vi "Actor Core.vi"(8 "error in":errorcluster, 11 "Import Export in":refnum<class "Import Export SQL.lvclass">) -> (0 "error out":errorcluster, 3 "Actor out":refnum<class "Actor.lvclass">)   [LabVIEW 2023, in "Data Analysis.lvlib" / "Import Export SQL.lvlib" / "Import Export SQL.lvclass"]
doc: "(<B>Filename</B>: Actor Framework.lvlib:Actor.lvclass:Actor Core.vi)\n\nReceives messages to the actor, reacts to them, and initiates any error handling that may shut the actor down.\n\nDescendant classes may override this VI to append parallel tasks for the actor to complete while it handles messages. Overrides use the Call Parent Class Method node."
uses:
  Import Export SQL.lvclass
  C:/Program Files/National Instruments/LabVIEW 2023/vi.lib/ActorFramework/Actor/Actor.lvclass
  <vilib>/ActorFramework/Actor/Actor.lvclass
  Import Export SQL.lvclass/Import Export SQL.ctl
  <vilib>/ActorFramework/Actor/Actor.lvclass/Actor.ctl
  <vilib>/ActorFramework/Message Enqueuer/Message Enqueuer.lvclass/Message Enqueuer.ctl
  Subpanel-Abstract Messages/Insert SP Msg/Insert SP Msg.lvclass/Insert SP Msg.ctl
  Import Export SQL Messages/Write Schema Name Msg/Write Schema Name Msg.lvclass/Write Schema Name Msg.ctl
  Import Export SQL Messages/Export SQL Msg/Export SQL Msg.lvclass/Export SQL Msg.ctl
  Import Export SQL Messages/Import SQL Msg/Import SQL Msg.lvclass/Import SQL Msg.ctl
  <vilib>/ActorFramework/Message Enqueuer/Init from Existing Queue.vi
  <vilib>/ActorFramework/Message Enqueuer/Enqueue.vi
  Subpanel-Abstract Messages/Insert SP Msg/Insert SP Msg.lvclass
  C:/Program Files/National Instruments/LabVIEW 2023/vi.lib/ActorFramework/Message/Message.lvclass
  Import Export SQL Messages/Show the Schemas Msg/Show the Schemas Msg.lvclass
  Import Export SQL Messages/Write Schema Name Msg/Write Schema Name Msg.lvclass
  Import Export SQL Messages/Export SQL Msg/Export SQL Msg.lvclass
  Import Export SQL Messages/Import SQL Msg/Import SQL Msg.lvclass
  <vilib>/ActorFramework/Message Priority Queue/Priority Enqueue.vi
  <vilib>/ActorFramework/Message Enqueuer/Message Enqueuer.lvclass
  Subpanel-Abstract/Subpanel-Abstract.lvclass
  D:/eDCU LTT/VT LTT Project/Source Code/Data Analysis/Subpanel-Abstract/Subpanel-Abstract.lvclass
  D:/eDCU LTT/VT LTT Project/Source Code/Data Analysis/Import Export SQL/Import Export/Import Export SQL.lvclass
panel:
  out "Status":string
  in  "Tab Control":enum32{"Import", "Export"}(tab)
  in  "Select the test log file to be imported(.sql)":path
  in  "Import Schema Name":string(combo) caption="Schema Name"
  in  "Import SQL":bool
  in  "Select the Folder":path
  in  "Export Schema Name":string(combo) caption="Test Log Name"
  in  "Export SQL":bool
  in  "Schema Names":string(combo)
  in  "Stop":bool
  # "One Combo Box- Show all the Tables for Selected Schema.\n2. Export Option Enable FE, FF Actor to"
  # "Export Data"
  # "*All filters are applicable here"
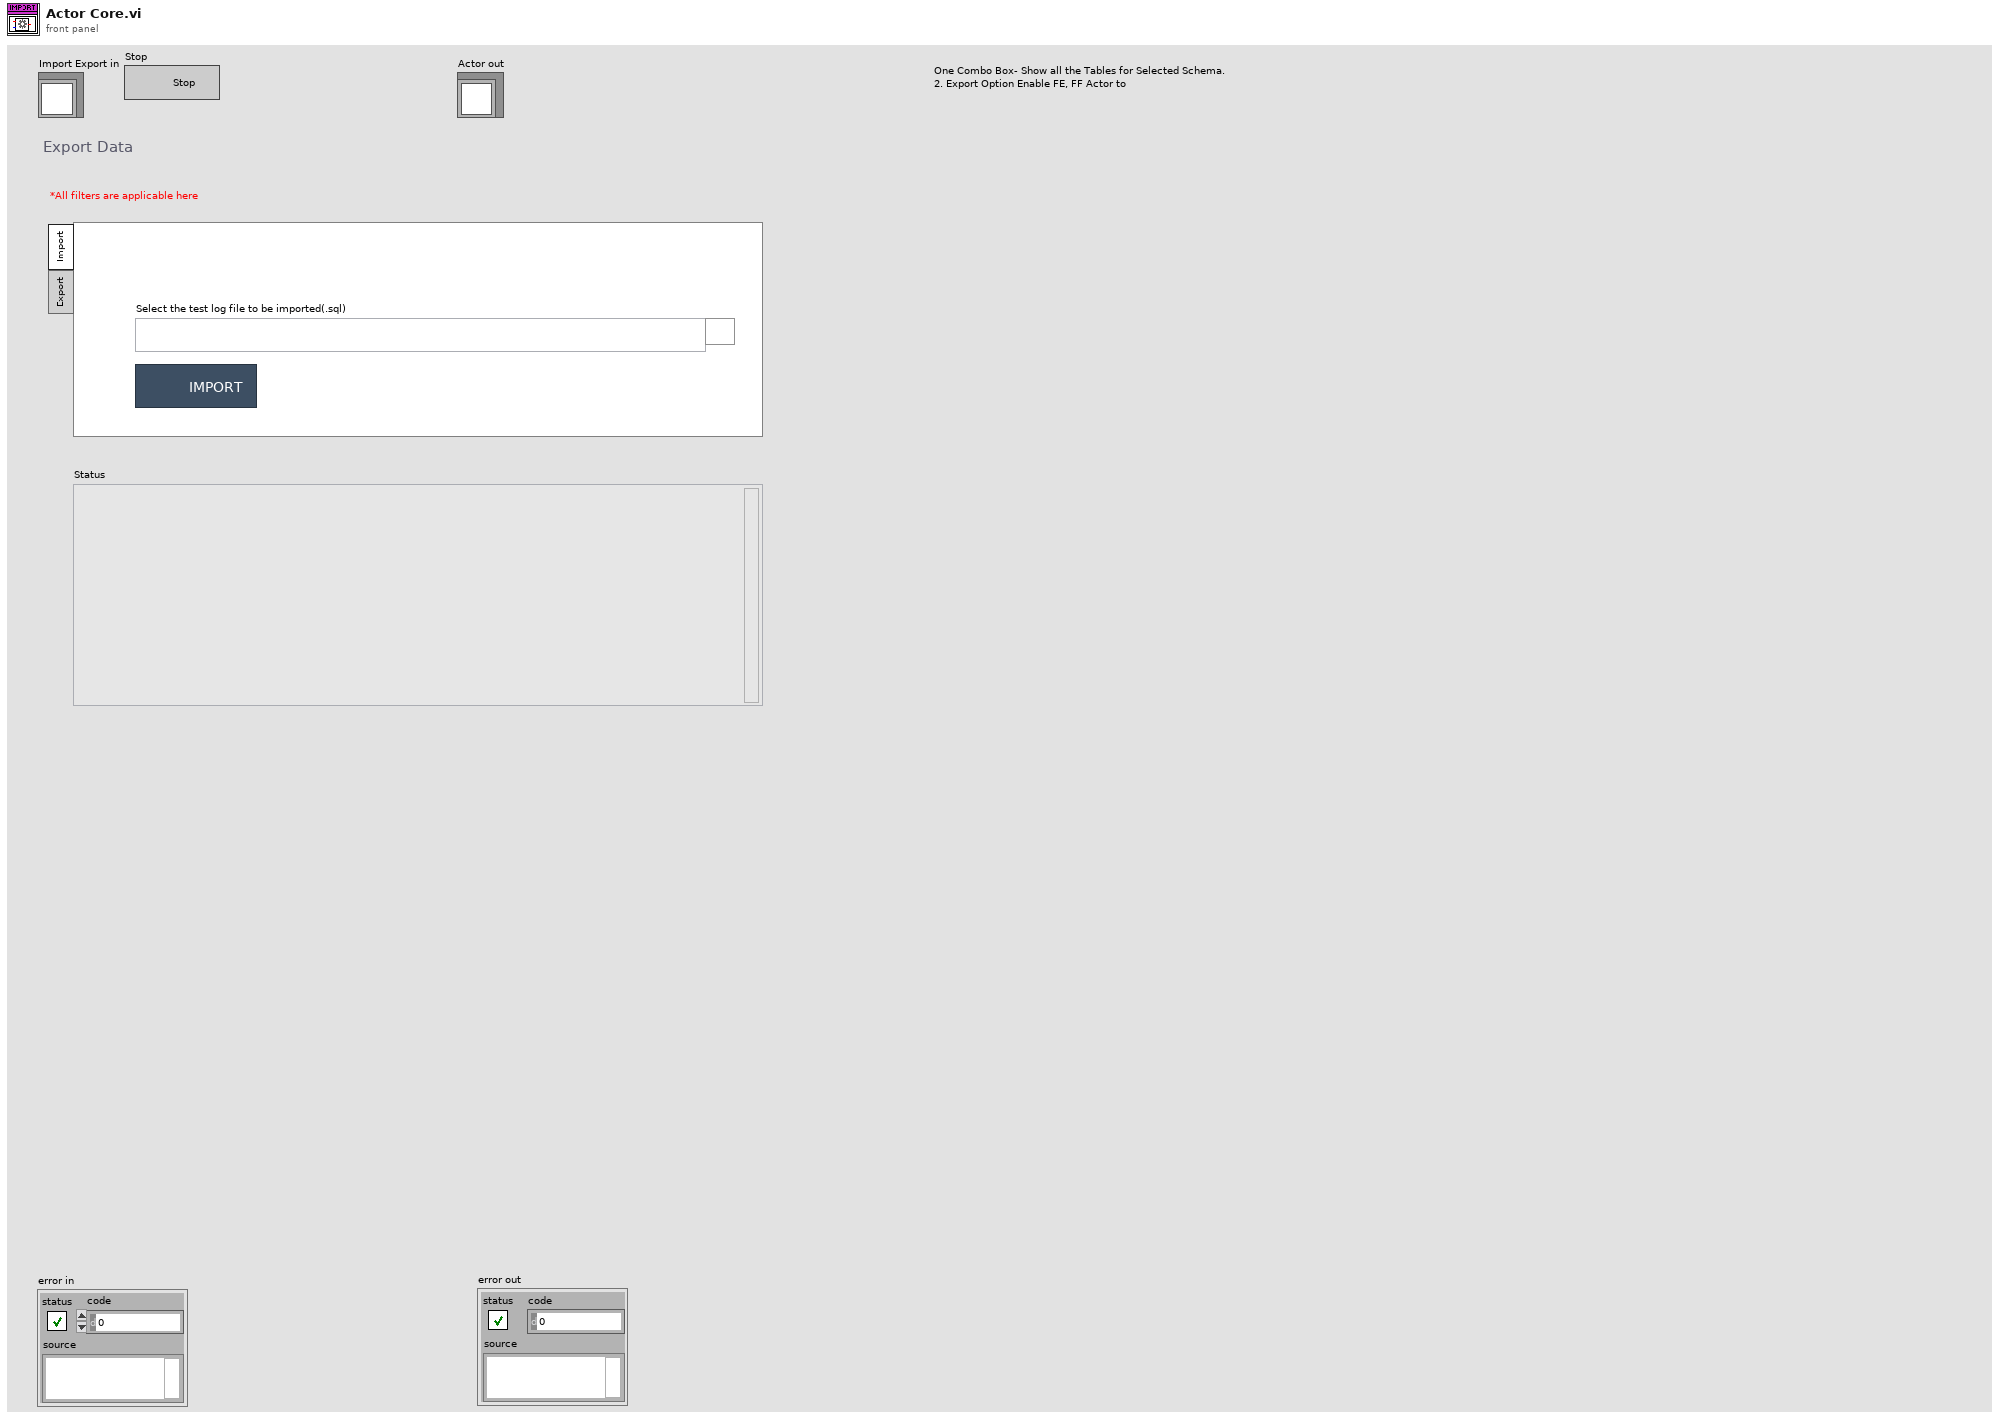
[diagram p1: front panel]
types:
  T1 = cluster{"Schema":string, "Save File Path":path, "Script File Path":path}
  T2 = cluster{"Schema Name":string, "Dump File Path":path, "Script Path":path}
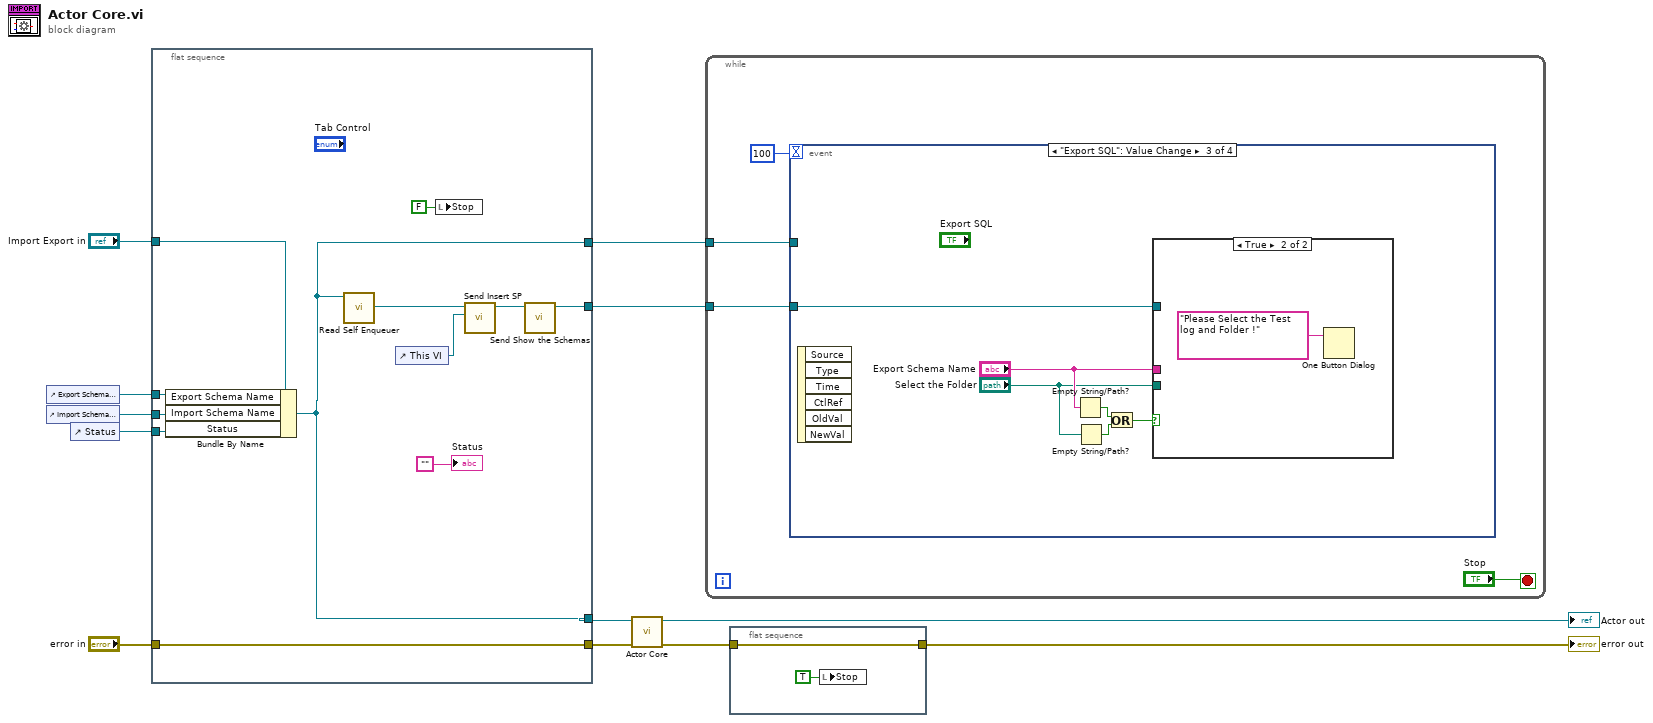
[diagram p0: block diagram]
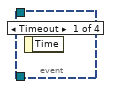
[diagram p2: hidden frame]
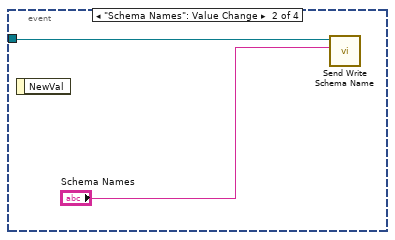
[diagram p3: hidden frame]
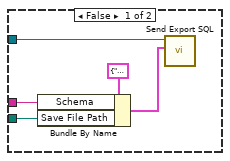
[diagram p4: hidden frame]
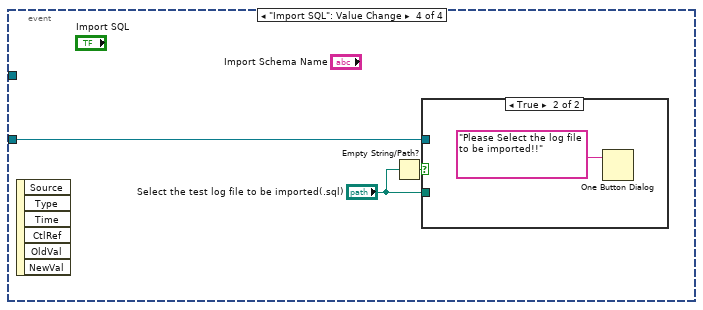
[diagram p5: hidden frame]
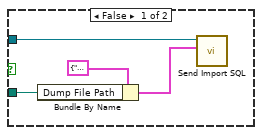
[diagram p6: hidden frame]
diagram:
  n1 = control-ref of="Export Schema Name"() -> (w3:refnum<vi>)
  n2 = control-ref of="Import Schema Name"() -> (w2:refnum<vi>)
  n3 = control-ref of="Status"() -> (w1:refnum<vi>)
  n4 = flat-sequence {
    tunnel: "error in" -> [w24]
    tunnel: [w24] -> w10
    tunnel: "Import Export in" -> [w20]
    tunnel: [w18] -> w8
    tunnel: [w16] -> w7
    tunnel: [w18] -> w6
    tunnel: w3 -> [w19]
    tunnel: w2 -> [w15]
    tunnel: w1 -> [w14]
    frame #0 {
      n5 = Bundle By Name(cluster=w20, "Export Schema Name"=w19, "Import Schema Name"=w15, "Status"=w14) -> (w18:refnum<class "Import Export SQL.lvclass">)
      n6 = call <vilib>:"Read Self Enqueuer.vi"("Actor"=w18) -> ("Self Enqueuer"=w22:refnum<class "Message Enqueuer.lvclass">)  [unwired: 10 in]
      n7 = control-ref of="This VI"() -> (w21:refnum<vi>)
      n8 = local write "Stop"(FALSE ("Stop")) -> ()
      n9 = call "Send Insert SP.vi"("VI Ref"=w21, "Message Enqueuer"=w22) -> ("Message Enqueuer out"=w17:refnum<class "Message Enqueuer.lvclass">)  [unwired: 8 in, 1 out]
      n10 = call "Send Show the Schemas.vi"("Message Enqueuer"=w17) -> ("Message Enqueuer out"=w16:refnum<class "Message Enqueuer.lvclass">)  [unwired: 9 in, 1 out]
      "Status" <- ""
    }
  }
  n11 = call-parent "Actor Core.vi"("error in"=w10, "Actor in"=w8) -> ("error out"=w5:errorcluster, "Actor out"=→"Actor out":refnum<class "Actor.lvclass">)  [unwired: 8 in]
  n12 = while {
    tunnel: w7 -> [w26]
    tunnel: w6 -> [w25]
    stop <- "Stop" stop-if-true
    n13 = event shown="[2] \"Export SQL\": Value Change" {
      selector: _ -> [_ _ _ _]
      dyn-events: _ -> [_ _ _ _]
      timeout: 100 -> [_ _ _ _]
      tunnel: w26 -> [_ w30 w36 w45]
      tunnel: w25 -> [_ _ _ _]
      event Timeout {
        n14 = event-data() -> ()  [unwired: 1 in, 1 out]
      }
      event "Schema Names": Value Change {
        n15 = event-data() -> ()  [unwired: 1 in, 1 out]
        n16 = call "Send Write Schema Name.vi"("Schema Name"="Schema Names", "Message Enqueuer"=w30) -> ()  [unwired: 8 in, 2 out]
      }
      event "Export SQL": Value Change {
        n17 = event-data() -> ()  [unwired: 1 in, 6 out]
        n18 = Empty String/Path?(string/path="Export Schema Name") -> (empty?=w35:bool)
        n19 = Empty String/Path?(string/path="Select the Folder") -> (empty?=w34:bool)
        n20 = Or(x=w35, y=w34) -> (x .or. y?=w31:bool)
        n21 = case shown="True" w31 {
          tunnel: w36 -> [w41 _]
          tunnel: "Export Schema Name" -> [w38 _]
          tunnel: "Select the Folder" -> [w37 _]
          frame False {
            n22 = Bundle By Name(cluster=T1 {"Schema"="", "Save File Path"=path "", "Script File Path"=path ""} ("Export Data"), "Schema"=w38, "Save File Path"=w37) -> (w39:T1)
            n23 = call "Send Export SQL.vi"("Export Data"=w39, "Message Enqueuer"=w41) -> ()  [unwired: 8 in, 2 out]
          }
          frame True {
            n24 = One Button Dialog(message="Please Select the Test log and Folder !") -> ()  [unwired: 1 in, 1 out]
          }
        }
      }
      event "Import SQL": Value Change {
        n25 = event-data() -> ()  [unwired: 1 in, 6 out]
        n26 = Empty String/Path?(string/path="Select the test log file to be imported(.sql)") -> (empty?=w43:bool)
        n27 = case shown="True" w43 {
          tunnel: w45 -> [w49 _]
          tunnel: "Select the test log file to be imported(.sql)" -> [w46 _]
          frame False {
            n28 = Bundle By Name(cluster=T2 {"Schema Name"="", "Dump File Path"=path "", "Script Path"=path ""} ("Import Data"), "Dump File Path"=w46) -> (w47:T2)
            n29 = call "Send Import SQL.vi"("Import Data"=w47, "Message Enqueuer"=w49) -> ()  [unwired: 8 in, 2 out]
          }
          frame True {
            n30 = One Button Dialog(message="Please Select the log file to be imported!!") -> ()  [unwired: 1 in, 1 out]
          }
        }
      }
    }
  }
  n31 = flat-sequence {
    tunnel: w5 -> [w52]
    tunnel: [w52] -> w4
    frame #0 {
      n32 = local write "Stop"(TRUE ("Stop")) -> ()
    }
  }
  "error out" <- w4
